vi "Configure Calibration Security1.vi"(8 "error in (no error)":errorcluster, 9 "Enable Security (T: Enable)":bool=TRUE, 10 "Security Code ()":string, 11 "VISA resource name":refnum<visa-resource-name>) -> (0 "error out":errorcluster, 3 "VISA resource name out":refnum<visa-resource-name>)   [LabVIEW 2015, in "Agilent 3446X Series1.lvlib"]
doc: "Configures security settings for calibration."
uses:
  Agilent 3446X Series1.lvlib
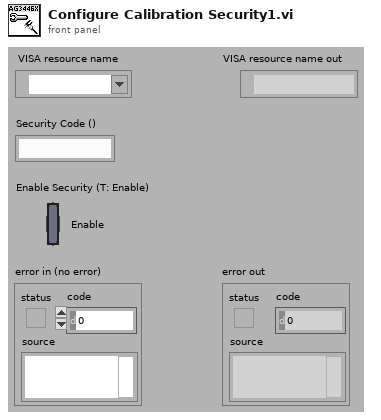
[diagram p1: front panel]
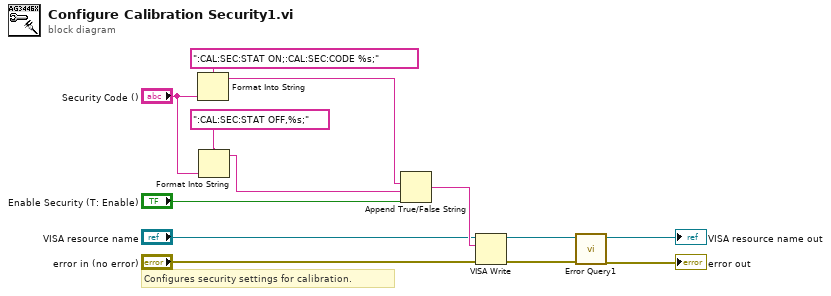
[diagram p0: block diagram]
diagram:
  # "Configures security settings for calibration."
  n1 = Format Into String(format string=":CAL:SEC:STAT ON;:CAL:SEC:CODE %s;", "Security Code ()") -> (resulting string=w4:string)  [unwired: 2 in, 1 out]
  n2 = Format Into String(format string=":CAL:SEC:STAT OFF,%s;", "Security Code ()") -> (resulting string=w1:string)  [unwired: 2 in, 1 out]
  n3 = Append True/False String(1:"Enable Security (T: Enable)", 2:w1, 3:w4) -> (0:w11:string)  [unwired: 1 out]
  n4 = VISA Write(VISA resource name="VISA resource name", write buffer=w11, error in (no error)="error in (no error)") -> (VISA resource name out=w8:refnum<visa-resource-name>, error out=w7:errorcluster)  [unwired: 1 out]
  n5 = call "Error Query1.vi"("error in (no error)"=w7, "VISA resource name"=w8) -> ("error out"=→"error out":errorcluster, "VISA resource name out"=→"VISA resource name out":refnum<visa-resource-name>)  [unwired: 8 out]
